vi "send response.vi"(6 "udp message":string, 7 "connection ID out":refnum<k16>, 8 "error in (no error)":errorcluster, 9 "port":u16, 10 "address":u32, 11 "UDP_transmitter in":refnum<class "UDP_transmitter.lvclass">) -> (0 "error out":errorcluster, 3 "UDP_transmitter out":refnum<class "UDP_transmitter.lvclass">)   [LabVIEW 2025, in "UDP_transmitter.lvlib" / "UDP_transmitter.lvclass"]
uses:
  UDP_transmitter.lvclass
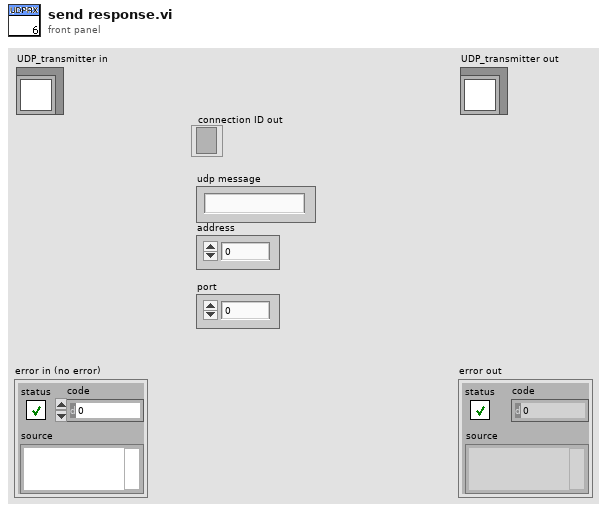
[diagram p1: front panel]
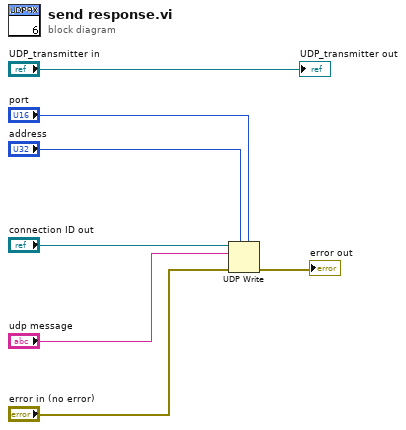
[diagram p0: block diagram]
diagram:
  n1 = UDP Write(address="address", port or service name="port", connection ID="connection ID out", data in="udp message", 8:"error in (no error)") -> (error out=→"error out":errorcluster)  [unwired: 1 in, 1 out]
  "UDP_transmitter out" <- "UDP_transmitter in"
